vi "DB Script.vi"() -> ()   [LabVIEW 2018]
panel:
  out "resulting string":string
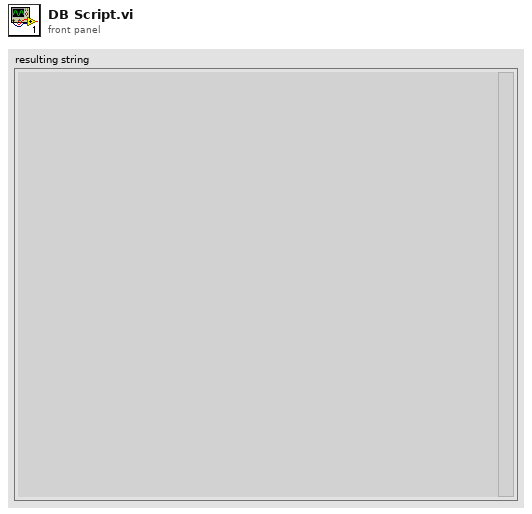
[diagram p1: front panel]
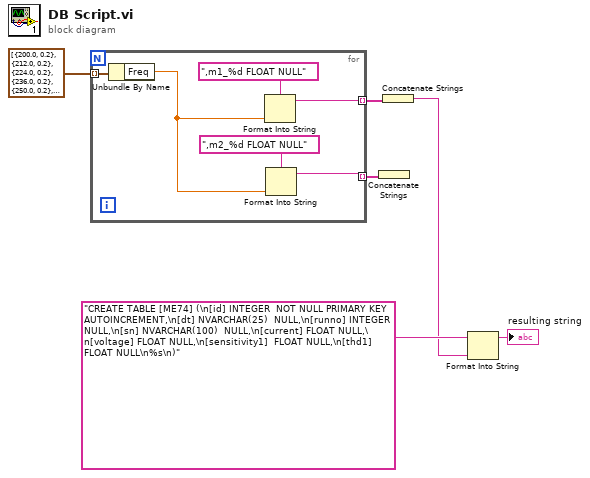
[diagram p0: block diagram]
diagram:
  n1 = for {
    tunnel: cluster{"Freq":dbl, "Amp":dbl}[] [{"Freq"=200.0, "Amp"=0.2}, {"Freq"=212.0, "Amp"=0.2}, {"Freq"=224.0, "Amp"=0.2}, {"Freq"=236.0, "Amp"=0.2}, {"Freq"=250.0, "Amp"=0.2}, {"Freq"=265.0, "Amp"=0.2}, {"Freq"=280.0, "Amp"=0.2}, {"Freq"=300.0, "Amp"=0.2}, {"Freq"=315.0, "Amp"=0.2}, {"Freq"=335.0, "Amp"=0.2}, {"Freq"=355.0, "Amp"=0.2}, {"Freq"=375.0, "Amp"=0.2}, {"Freq"=400.0, "Amp"=0.2}, {"Freq"=425.0, "Amp"=0.2}, {"Freq"=450.0, "Amp"=0.2}, {"Freq"=475.0, "Amp"=0.2}, {"Freq"=500.0, "Amp"=0.2}, {"Freq"=530.0, "Amp"=0.2}, {"Freq"=560.0, "Amp"=0.2}, {"Freq"=600.0, "Amp"=0.2}, {"Freq"=630.0, "Amp"=0.2}, {"Freq"=670.0, "Amp"=0.2}, {"Freq"=710.0, "Amp"=0.2}, {"Freq"=750.0, "Amp"=0.2}, {"Freq"=800.0, "Amp"=0.2}, {"Freq"=850.0, "Amp"=0.2}, {"Freq"=900.0, "Amp"=0.2}, {"Freq"=950.0, "Amp"=0.2}, {"Freq"=1000.0, "Amp"=0.2}, {"Freq"=1060.0, "Amp"=0.2}, {"Freq"=1120.0, "Amp"=0.2}, {"Freq"=1180.0, "Amp"=0.2}, {"Freq"=1250.0, "Amp"=0.2}, {"Freq"=1320.0, "Amp"=0.2}, {"Freq"=1400.0, "Amp"=0.2}, {"Freq"=1500.0, "Amp"=0.2}, {"Freq"=1600.0, "Amp"=0.2}, {"Freq"=1700.0, "Amp"=0.2}, {"Freq"=1800.0, "Amp"=0.2}, {"Freq"=1900.0, "Amp"=0.2}, {"Freq"=2000.0, "Amp"=0.2}, {"Freq"=2120.0, "Amp"=0.2}, {"Freq"=2240.0, "Amp"=0.2}, {"Freq"=2360.0, "Amp"=0.2}, {"Freq"=2500.0, "Amp"=0.2}, {"Freq"=2650.0, "Amp"=0.2}, {"Freq"=2800.0, "Amp"=0.2}, {"Freq"=3000.0, "Amp"=0.2}, {"Freq"=3150.0, "Amp"=0.2}, {"Freq"=3350.0, "Amp"=0.2}, {"Freq"=3550.0, "Amp"=0.2}, {"Freq"=3750.0, "Amp"=0.2}, {"Freq"=4000.0, "Amp"=0.2}, {"Freq"=4250.0, "Amp"=0.2}, {"Freq"=4500.0, "Amp"=0.2}, {"Freq"=4750.0, "Amp"=0.2}, {"Freq"=5000.0, "Amp"=0.2}, {"Freq"=5300.0, "Amp"=0.2}, {"Freq"=5600.0, "Amp"=0.2}, {"Freq"=6000.0, "Amp"=0.2}, {"Freq"=6300.0, "Amp"=0.2}, {"Freq"=6700.0, "Amp"=0.2}, {"Freq"=7100.0, "Amp"=0.2}, {"Freq"=7500.0, "Amp"=0.2}, {"Freq"=8000.0, "Amp"=0.2}] ("Freq List In") -> [w12] mode=indexing
    tunnel: [w10] -> w5 mode=indexing
    tunnel: [w7] -> w1 mode=indexing
    n2 = Unbundle By Name(w12) -> ("Freq"=w8:dbl)
    n3 = Format Into String(format string=",m1_%d FLOAT NULL", w8) -> (resulting string=w10:string)  [unwired: 2 in, 1 out]
    n4 = Format Into String(format string=",m2_%d FLOAT NULL", w8) -> (resulting string=w7:string)  [unwired: 2 in, 1 out]
  }
  n5 = Concatenate Strings(w1) -> ()  [unwired: 1 out]
  n6 = Concatenate Strings(w5) -> (w3:string)
  n7 = Format Into String(format string="CREATE TABLE [ME74] (\n[id] INTEGER  NOT NULL PRIMARY KEY AUTOINCREMENT,\n[dt] NVARCHAR(25)  NULL,\n[runno] INTEGER  NULL,\n[sn] NVARCHAR(100)  NULL,\n[current] FLOAT NULL,\n[voltage] FLOAT NULL,\n[sensitivity1]  FLOAT NULL,\n[thd1] FLOAT NULL\n%s\n)", w3) -> (resulting string=→"resulting string":string)  [unwired: 2 in, 1 out]
